vi "Time_String_to_Stamp.vi"(11 "Published Data":string[][](array[string])) -> (2 "time stamp":timestamp, 3 "Values":dbl[](array[numeric]))   [LabVIEW 2015]
uses:
  <vilib>/Utility/miscctls.llb/LVDateTimeRec.ctl
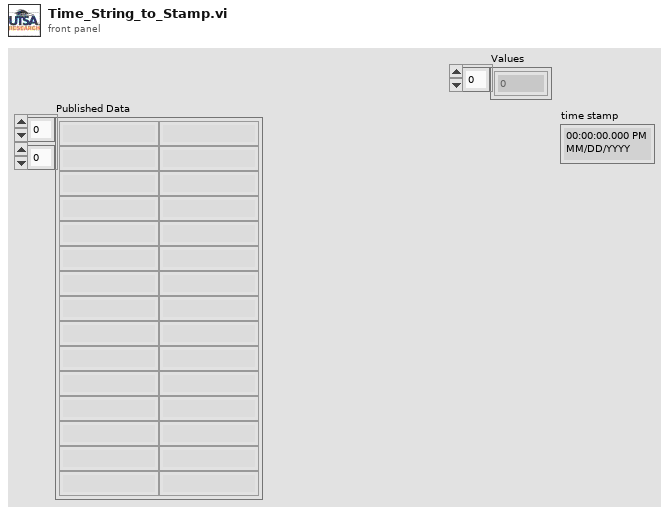
[diagram p1: front panel]
types:
  T1 = typedef "LVDateTimeRec.ctl" = cluster{"fractional second":dbl, "second":i32, "minute":i32, "hour":i32, "day of month":i32, "month":i32, "year":i32, "day of week":i32, "day of year":i32, "DST":i32}
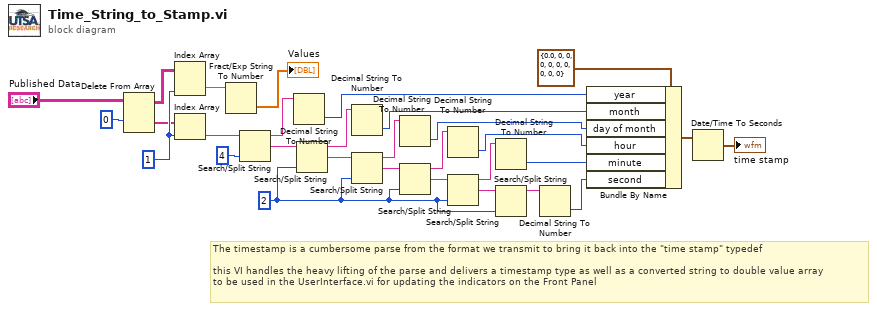
[diagram p0: block diagram]
diagram:
  w13 = 2 ("offset (0)")
  w27 = 1 ("index")
  # "The timestamp is a cumbersome parse from the format we transmit to bring it back into the \"time stamp\" typedef\n\nthis VI handles the heavy lifting of the parse and delivers a timestamp type as well as a converted string to double value array\nto be used in the UserInterface.vi for updating the indicators on the Front Panel"
  n1 = Delete From Array(array="Published Data", index (row)=0 ("length")) -> (deleted portion=w6:string[], array with subset deleted=w4:string[][])  [unwired: 2 in]
  n2 = Index Array(array=w4, index (col)=w27) -> (element=w2:string[])  [unwired: 1 in]
  n3 = Index Array(array=w6, index=w27) -> (element=w7:string)
  n4 = Fract/Exp String To Number(string=w2) -> (number=→"Values":dbl[])  [unwired: 3 in, 1 out]
  n5 = Search/Split String(string=w7, offset (0)=4) -> (substring before match=w21:string, match + rest of string=w9:string)  [unwired: 1 in, 1 out]
  n6 = Decimal String To Number(string=w21) -> (number=w15:i32)  [unwired: 2 in, 1 out]
  n7 = Search/Split String(string=w9, offset (0)=w13) -> (substring before match=w22:string, match + rest of string=w10:string)  [unwired: 1 in, 1 out]
  n8 = Decimal String To Number(string=w22) -> (number=w16:i32)  [unwired: 2 in, 1 out]
  n9 = Search/Split String(string=w10, offset (0)=w13) -> (substring before match=w23:string, match + rest of string=w11:string)  [unwired: 1 in, 1 out]
  n10 = Decimal String To Number(string=w23) -> (number=w17:i32)  [unwired: 2 in, 1 out]
  n11 = Search/Split String(string=w11, offset (0)=w13) -> (substring before match=w24:string, match + rest of string=w12:string)  [unwired: 1 in, 1 out]
  n12 = Decimal String To Number(string=w24) -> (number=w18:i32)  [unwired: 2 in, 1 out]
  n13 = Search/Split String(string=w12, offset (0)=w13) -> (substring before match=w25:string, match + rest of string=w14:string)  [unwired: 1 in, 1 out]
  n14 = Decimal String To Number(string=w25) -> (number=w19:i32)  [unwired: 2 in, 1 out]
  n15 = Search/Split String(string=w14, offset (0)=w13) -> (substring before match=w26:string)  [unwired: 1 in, 2 out]
  n16 = Decimal String To Number(string=w26) -> (number=w20:i32)  [unwired: 2 in, 1 out]
  n17 = Bundle By Name(cluster=T1 {"fractional second"=0.0, "second"=0, "minute"=0, "hour"=0, "day of month"=0, "month"=0, "year"=0, "day of week"=0, "day of year"=0, "DST"=0} ("date time rec"), "year"=w15, "month"=w16, "day of month"=w17, "hour"=w18, "minute"=w19, "second"=w20) -> (w30:T1)
  n18 = Date/Time To Seconds(2:w30) -> (0:→"time stamp":timestamp)  [unwired: 1 in]
